vi "Actor Core.vi"(8 "error in":errorcluster, 11 "Elevator Controller in":refnum<class "Sim User Console Actor.lvclass">) -> (0 "error out":errorcluster, 3 "Actor out":refnum<class "Actor.lvclass">)   [LabVIEW 2019, in "Sim User Console Actor.lvlib" / "Sim User Console Actor.lvclass"]
doc: "(<B>Filename</B>: Actor Framework.lvlib:Actor.lvclass:Actor Core.vi)\n\nReceives messages to the actor, reacts to them, and initiates any error handling that may shut the actor down.\n\nDescendant classes may override this VI to append parallel tasks for the actor to complete while it handles messages. Overrides use the Call Parent Method node."
uses:
  Sim User Console Actor.lvclass
  <vilib>/ActorFramework/Actor/Actor.lvclass
  <vilib>/ActorFramework/Stop Msg/Stop Msg.lvclass
  Elevator Controller/Elevator Controller Messages/Set Floor Request Msg/Set Floor Request Msg.lvclass
  C:/Workspace/CLA/Elevator AF 3rd/User Console Actor/User Console Actor/User Console Actor.lvclass
  C:/Program Files (x86)/National Instruments/LabVIEW 2019/vi.lib/ActorFramework/Actor/Actor.lvclass
  Elevator Controller/Elevator Controller Messages/Set Elevator Call Request Msg/Set Elevator Call Request Msg.lvclass
  Elevator Controller/Elevator Controller Messages/Set Emergency Msg/Set Emergency Msg.lvclass
  Elevator Controller/Elevator Controller Messages/Wait for First Request Msg/Wait for First Request Msg.lvclass
  Elevator Controller/Elevator Controller Messages/Set Timing to 1 second Msg/Set Timing to 1 second Msg.lvclass
  User Console Actor/User Console Actor/User Console Actor.lvclass
  Elevator Controller/Elevator Controller Messages/Restart time Msg/Restart time Msg.lvclass
  Elevator Call -Cluster.ctl
  Floor Selection -Cluster.ctl
  Doors -Button.ctl
panel:
  in  "Emergency":bool
  in  "Door Buttons":T1
  in  "Floor Selection":T2
  in  "Elevator Call":T3
  # "[Covers: UI1]"
  # "[Covers: UI2A] \n[Covers: UI2A1]"
  # "[Covers: UI2]"
  # "[Covers: UI2B] \n[Covers: UI2B1]"
  # "[Covers: UI2C] \n[Covers: UI2C1] \n[Covers: UI2C2] \n[Covers: UI2C3]"
  # "[Covers: UI2D] \n[Covers: UI2D1]"
  # "Fourth Floor"
  # "Third Floor"
  # "Second Floor"
  # "First Floor"
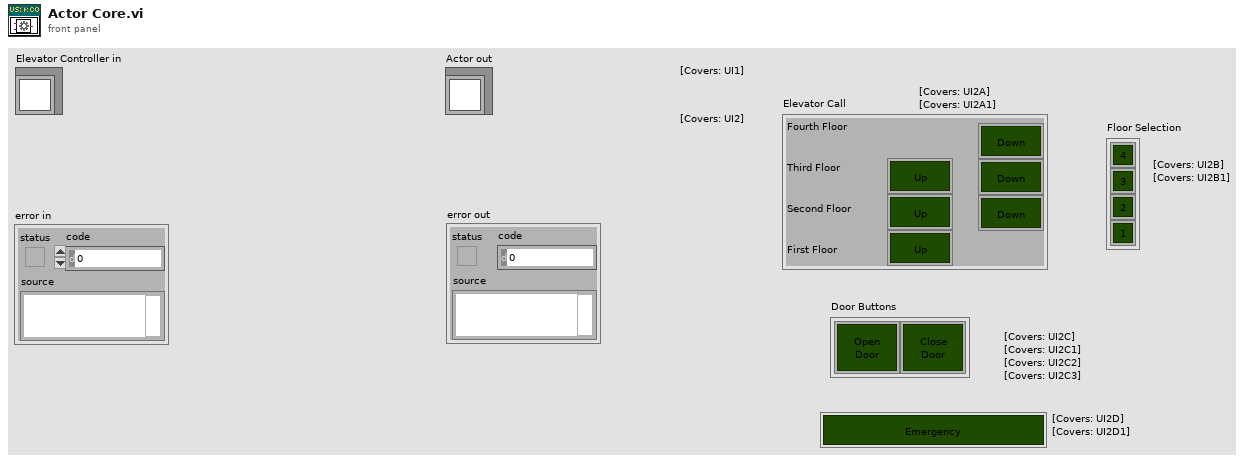
[diagram p1: front panel]
types:
  T1 = typedef "Sim User Console Actor.lvlib/Sim User Console Actor.lvclass/Doors -Button.ctl" = cluster{"Open Door":bool, "Close Door":bool}
  T2 = typedef "Sim User Console Actor.lvlib/Sim User Console Actor.lvclass/Floor Selection -Cluster.ctl" = cluster{"4":bool, "3":bool, "2":bool, "1":bool}
  T3 = typedef "Sim User Console Actor.lvlib/Sim User Console Actor.lvclass/Elevator Call -Cluster.ctl" = cluster{"Up 3":bool, "Up 2":bool, "Up 1":bool, "Down 4":bool, "Down 3":bool, "Down 2":bool}
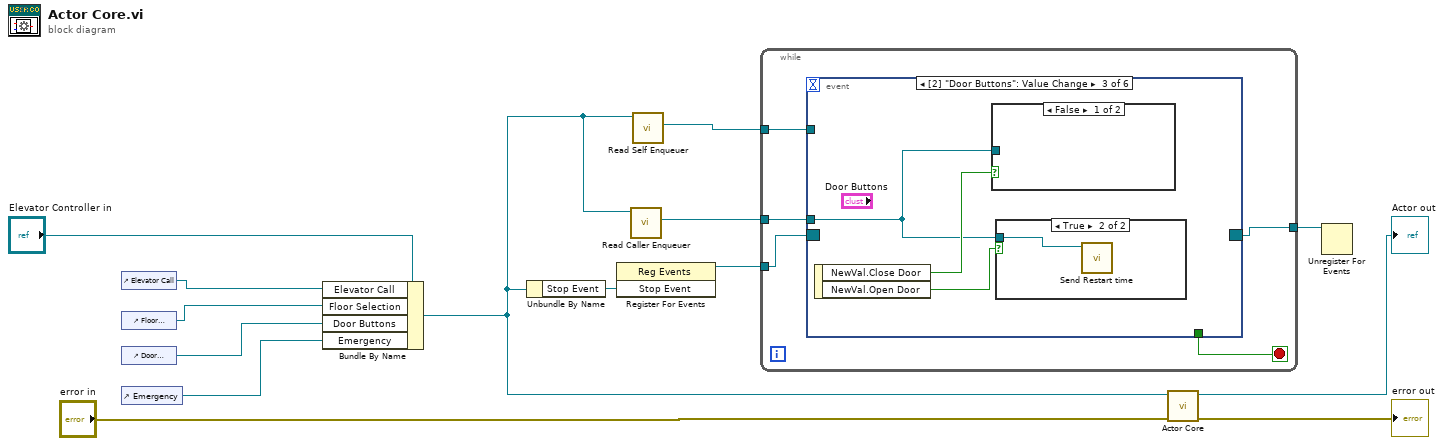
[diagram p0: block diagram]
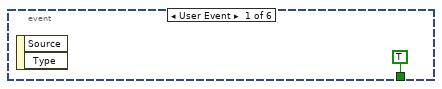
[diagram p2: hidden frame]
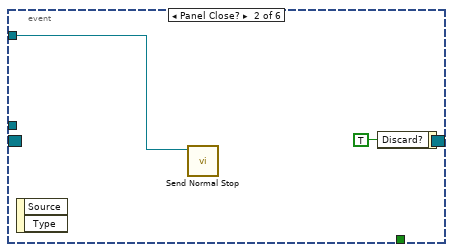
[diagram p3: hidden frame]
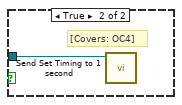
[diagram p5: hidden frame]
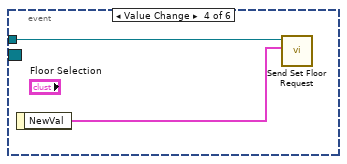
[diagram p6: hidden frame]
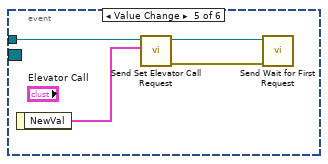
[diagram p7: hidden frame]
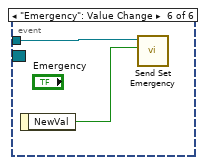
[diagram p8: hidden frame]
diagram:
  n1 = control-ref of="Elevator Call"() -> (w6:refnum<vi>)
  n2 = control-ref of="Floor Selection"() -> (w5:refnum<vi>)
  n3 = control-ref of="Door Buttons"() -> (w4:refnum<vi>)
  n4 = control-ref of="Emergency"() -> (w3:refnum<vi>)
  n5 = Bundle By Name(cluster="Elevator Controller in", "Elevator Call"=w6, "Floor Selection"=w5, "Door Buttons"=w4, "Emergency"=w3) -> (w2:refnum<class "Sim User Console Actor.lvclass">)
  n6 = Unbundle By Name(w2) -> ("Stop Event"=w9:refnum<user-event>)
  n7 = register-events(w9) -> (reference out=w11:refnum<event-registration>)  [unwired: 2 in, 1 out]
  n8 = call <vilib>:"Read Caller Enqueuer.vi"("Actor"=w2) -> ("Caller Enqueuer"=w1:refnum<class "Message Enqueuer.lvclass">)  [unwired: 10 in]
  n9 = call <vilib>:"Read Self Enqueuer.vi"("Actor"=w2) -> ("Self Enqueuer"=w8:refnum<class "Message Enqueuer.lvclass">)  [unwired: 10 in]
  n10 = while {
    tunnel: w11 -> [w19]
    tunnel: [w18] -> w10
    tunnel: w8 -> [w17]
    tunnel: w1 -> [w15]
    stop <- w16 stop-if-true
    n11 = event shown="[2] \"Door Buttons\": Value Change" {
      selector: w19 -> [_ _ _ _ _ _]
      dyn-events: [_ _ _ _ _ _] -> w18
      timeout: _ -> [_ _ _ _ _ _]
      tunnel: w17 -> [_ w21 _ _ _ _]
      tunnel: [TRUE _ _ _ _ _] -> w16
      tunnel: w15 -> [_ _ w23 w28 w33 w35]
      event User Event {
        n12 = event-data() -> ()  [unwired: 1 in, 2 out]
      }
      event Panel Close? {
        n13 = event-data() -> ()  [unwired: 1 in, 2 out]
        n14 = call <vilib>:"Send Normal Stop.vi"("Message Enqueuer"=w21) -> ()  [unwired: 10 in, 1 out]
        n15 = event-data("Discard?"=TRUE) -> ()  [unwired: 1 in, 1 out]
      }
      event Value Change {
        n16 = event-data() -> ("NewVal.Close Door"=w25:bool, "NewVal.Open Door"=w24:bool)  [unwired: 1 in]
        n17 = case shown="False" w25 {
          tunnel: w23 -> [_ w27]
          frame False {
          }
          frame True {
            # "[Covers: OC4]"
            n18 = call "Send Set Timing to 1 second.vi"("Message Enqueuer"=w27) -> ()  [unwired: 9 in, 2 out]
          }
        }
        n19 = case shown="True" w24 {
          tunnel: w23 -> [_ w26]
          frame False {
          }
          frame True {
            n20 = call "Send Restart time.vi"("Message Enqueuer"=w26) -> ()  [unwired: 9 in, 2 out]
          }
        }
      }
      event Value Change {
        n21 = event-data() -> ("NewVal"=w29:T2)  [unwired: 1 in]
        n22 = call "Send Set Floor Request.vi"("Floor Selection"=w29, "Message Enqueuer"=w28) -> ()  [unwired: 8 in, 2 out]
      }
      event Value Change {
        n23 = event-data() -> ("NewVal"=w32:T3)  [unwired: 1 in]
        n24 = call "Send Set Elevator Call Request.vi"("Elevator Call"=w32, "Message Enqueuer"=w33) -> ("error out"=w31:errorcluster, "Message Enqueuer out"=w30:refnum<class "Message Enqueuer.lvclass">)  [unwired: 8 in]
        n25 = call "Send Wait for First Request.vi"("error in (no error)"=w31, "Message Enqueuer"=w30) -> ()  [unwired: 8 in, 2 out]
      }
      event "Emergency": Value Change {
        n26 = event-data() -> ("NewVal"=w34:bool)  [unwired: 1 in]
        n27 = call "Send Set Emergency.vi"("Emergency"=w34, "Message Enqueuer"=w35) -> ()  [unwired: 8 in, 2 out]
      }
    }
  }
  n28 = call-parent "Actor Core.vi"("error in"="error in", "Actor in"=w2) -> ("error out"=→"error out":errorcluster, "Actor out"=→"Actor out":refnum<class "Actor.lvclass">)  [unwired: 8 in]
  n29 = Unregister For Events(event registration refnum=w10) -> ()  [unwired: 1 in, 1 out]
